vi "create function16.vi"(6 "pApp":u32, 7 "eTextRep":i32, 8 "error in (no error)":errorcluster, 9 "nArg":i32, 10 "zFunctionName":u32, 11 "db":dbl) -> (0 "error out":errorcluster, 2 "function return":i32, 3 "db out":dbl, 4 "pApp out":u32)   [LabVIEW 2020, in "sqlite3.lvlib"]
uses:
  sqlite3.lvlib
  errstr.vi
  bin/sqlite3_64.dll
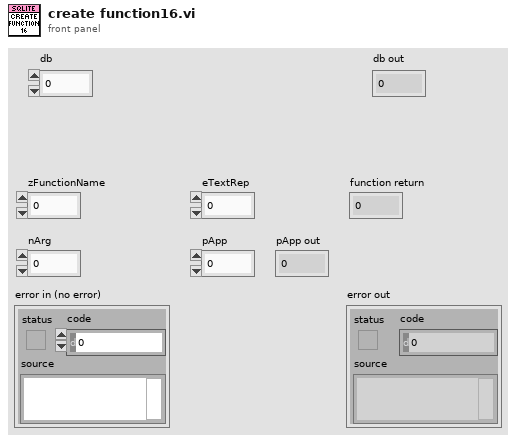
[diagram p1: front panel]
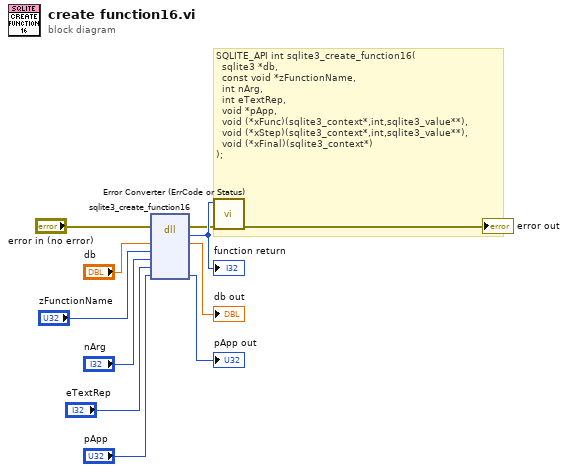
[diagram p0: block diagram]
diagram:
  # "SQLITE_API int sqlite3_create_function16(\n  sqlite3 *db,\n  const void *zFunctionName,\n  int nArg,\n  int eTextRep,\n  void *pApp,\n  void (*xFunc)(sqlite3_context*,int,sqlite3_value**),\n  void (*xStep)(sqlite3_context*,int,sqlite3_value**),\n  void (*xFinal)(sqlite3_context*)\n);"
  n1 = dll-call lib="C:/Users/Fred.Guo/Desktop/Database-configuration/externals/sqlite3/Source/bin/sqlite3_*.*" fn="sqlite3_create_function16"(error in="error in (no error)", "db"="db", "zFunctionName"="zFunctionName", "nArg"="nArg", "eTextRep"="eTextRep", "pApp"="pApp") -> (error out=w2:errorcluster, w11:i32, "db"=→"db out":dbl, "pApp"=→"pApp out":u32)  [unwired: 5 in, 1 out]
  "function return" <- w11
  n2 = call "Error Converter (ErrCode or Status).vi"("error in (no error)"=w2, "error code"=w11) -> ("error out"=→"error out":errorcluster)  [unwired: 9 in]
